vi "Schedule Geode Robot.vi"(6 "max geodes in":u8=24, 7 "max time in":u8=24, 8 "costs in":T1, 9 "data value reference":refnum<data-value>, 10 "stack in":refnum<queue>, 11 "mine in":refnum<class "Mine.lvclass">) -> (0 "costs out":T1, 1 "data value reference":refnum<data-value>, 2 "stack out":refnum<queue>, 3 "mine out":refnum<class "Mine.lvclass">, 4 "max geodes out":u8, 5 "max time out":u8)   [LabVIEW 2023, in "d19.lvlib" / "Mine.lvclass"]
uses:
  Mine.lvclass
  Mine.lvclass/Mine.ctl
  <vilib>/Utility/miscctls.llb/LVMapReplaceAction.ctl
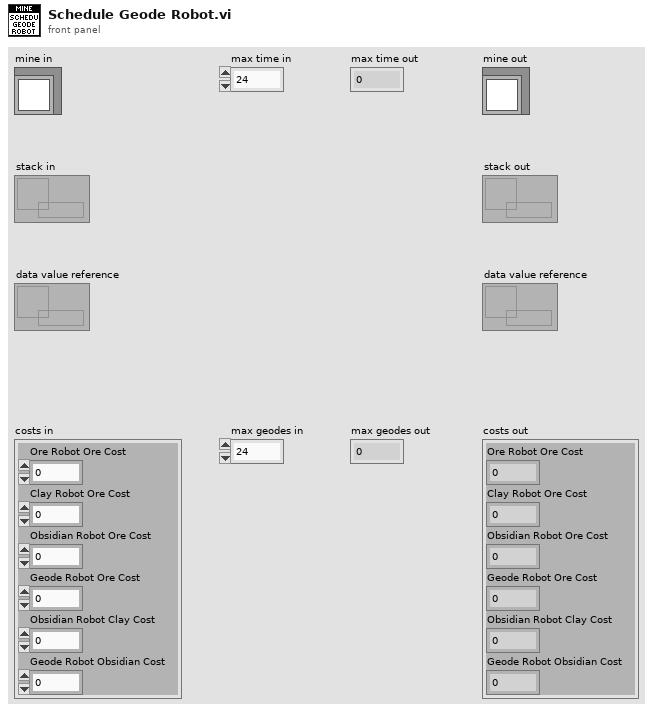
[diagram p1: front panel]
types:
  T1 = cluster{"Ore Robot Ore Cost":u8, "Clay Robot Ore Cost":u8, "Obsidian Robot Ore Cost":u8, "Geode Robot Ore Cost":u8, "Obsidian Robot Clay Cost":u8, "Geode Robot Obsidian Cost":u8}
  T2 = typedef "LVMapReplaceAction.ctl" = enum32{"Modify Entry only if found", "Add or Modify Entry", "Delete Entry"}
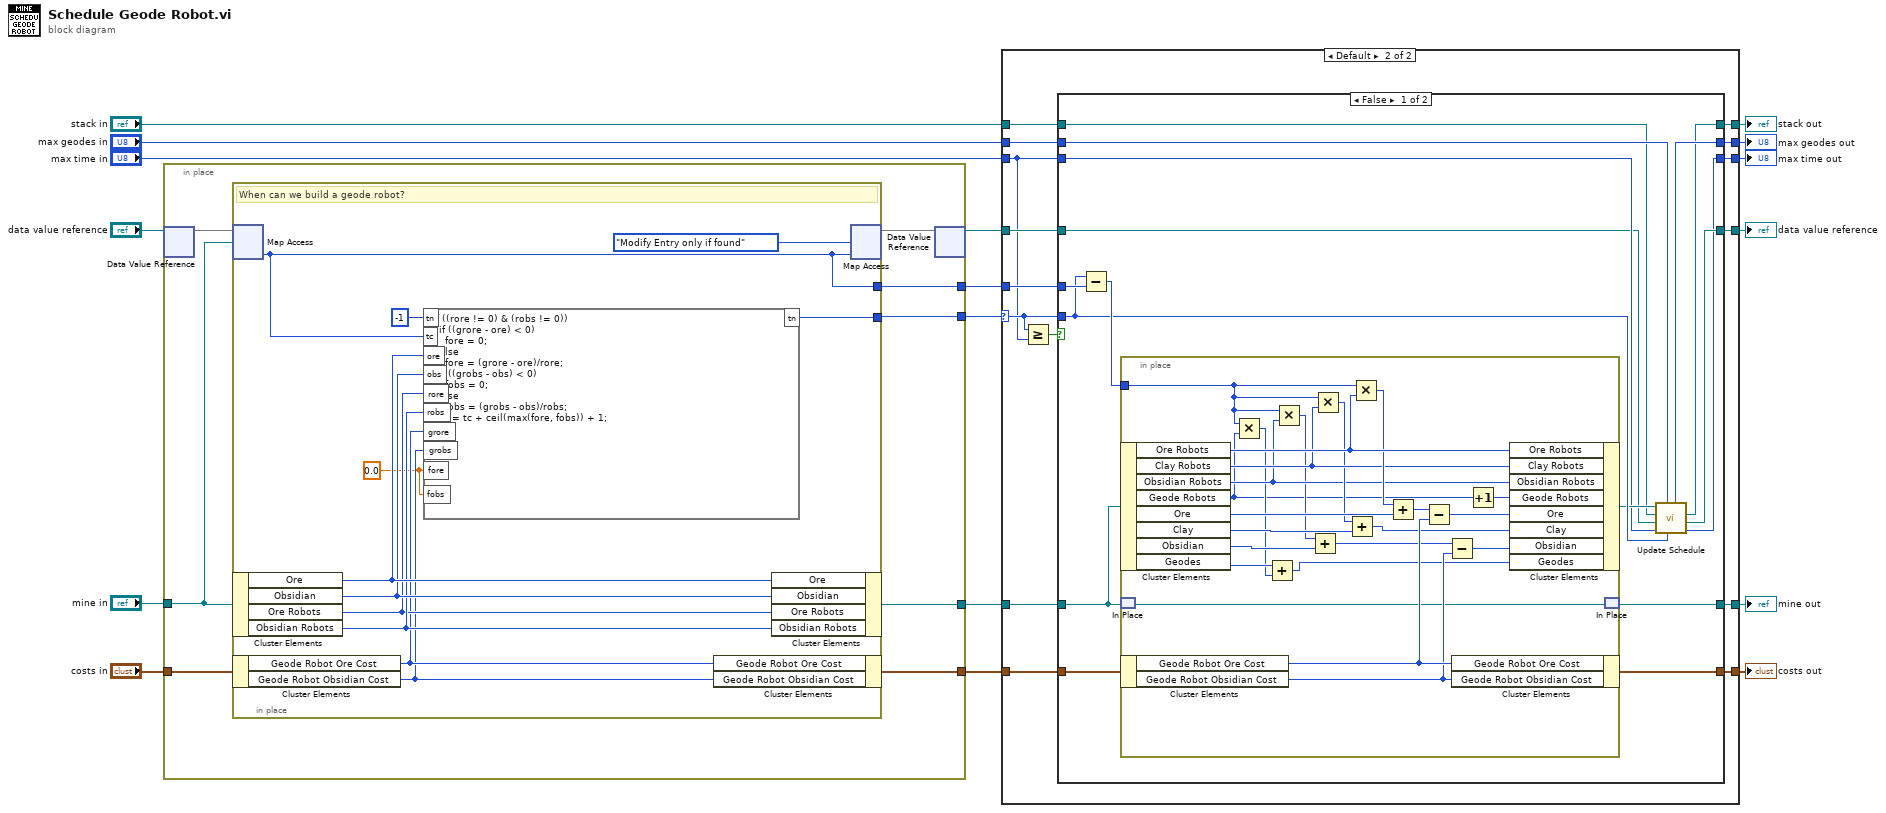
[diagram p0: block diagram]
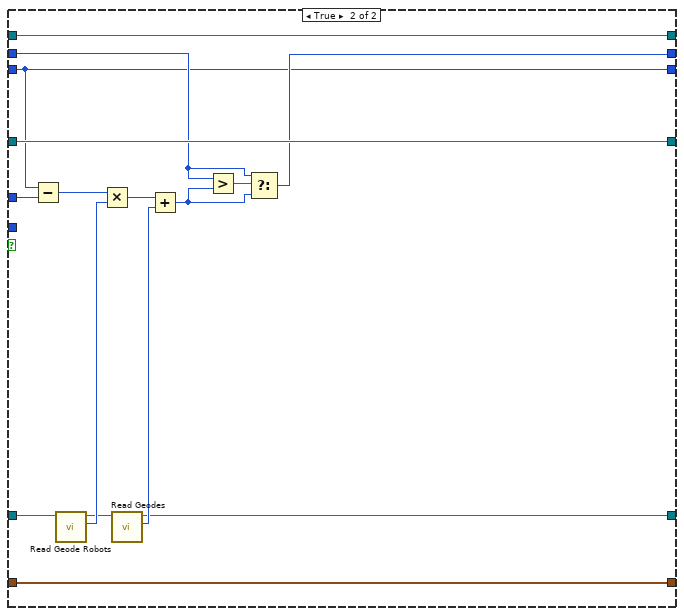
[diagram p3: hidden frame]
diagram:
  n1 = in-place {
    in-place-border: "costs in" -> [w25]
    in-place-border: "mine in" -> [w24]
    in-place-border: [w23] -> w15
    in-place-border: [w22] -> w11
    in-place-border: [w21] -> w10
    in-place-border: [w20] -> w6
    n2 = in-place-dvr #1("data value reference") -> (w19:map{refnum<class "Mine.lvclass">, u8})  [unwired: 1 out]
    n3 = in-place {
      in-place-border: [w28] -> w23
      in-place-border: [w26] -> w20
      w27 = 0.0 ("input variable")
      # "When can we build a geode robot?"
      n4 = in-place-map #2(w19, w24) -> (w26:u8)  [unwired: 1 in, 1 out]
      n5 = in-place-cluster #3(w24) -> ("Ore"=w35:u8, "Obsidian"=w34:u8, "Ore Robots"=w32:u8, "Obsidian Robots"=w33:u8)
      n6 = in-place-cluster #4(w25) -> ("Geode Robot Ore Cost"=w31:u8, "Geode Robot Obsidian Cost"=w30:u8)
      n7 = formula code="if ((rore != 0) & (robs != 0))\n  if ((grore - ore) < 0)\n    fore = 0;\n  else\n    fore = (grore - ore)/rore;\n  if ((grobs - obs) < 0)\n    fobs = 0;\n  else\n    fobs = (grobs - obs)/robs;\n  tn = tc + ceil(max(fore, fobs)) + 1;"("tc"=w26, "grore"=w31, "grobs"=w30, "ore"=w35, "obs"=w34, "rore"=w32, "robs"=w33, "tn"=i8 -1, "fore"=w27, "fobs"=w27) -> ("tn"=w28:i8)
      n8 = in-place-cluster #4("Geode Robot Ore Cost"=w31, "Geode Robot Obsidian Cost"=w30) -> (w22:T1)
      n9 = in-place-cluster #3("Ore"=w35, "Obsidian"=w34, "Ore Robots"=w32, "Obsidian Robots"=w33) -> (w21:refnum<class "Mine.lvclass">)
      n10 = in-place-map #2(w26, LVMapReplaceAction."Modify Entry only if found" ("action")) -> (w18:map{refnum<class "Mine.lvclass">, u8})  [unwired: 2 out]
    }
    n11 = in-place-dvr #1(w18) -> (w1:refnum<data-value>)  [unwired: 1 out]
  }
  n12 = case shown="Default" w15 {
    selector: w15 -> [_ w45]
    tunnel: "stack in" -> [w42 w57]
    tunnel: [w42 w56] -> w13
    tunnel: [w39 w55] -> w12
    tunnel: w11 -> [w37 w54]
    tunnel: w10 -> [w38 w53]
    tunnel: [w37 w52] -> w9
    tunnel: [w38 w51] -> w8
    tunnel: "max time in" -> [w40 w44]
    tunnel: w6 -> [_ w50]
    tunnel: "max geodes in" -> [w41 w49]
    tunnel: [w41 w48] -> w4
    tunnel: [w40 w47] -> w3
    tunnel: w1 -> [w39 w46]
    frame -1 {
    }
    frame Default {
      n13 = Greater Or Equal?(x=w45, y=w44) -> (x >= y?=w43:bool)
      n14 = case shown="False" w43 {
        tunnel: w46 -> [w62 w112]
        tunnel: [w60 w112] -> w55
        tunnel: w57 -> [w61 w111]
        tunnel: [w59 w111] -> w56
        tunnel: w54 -> [w73 w110]
        tunnel: w53 -> [w69 w99]
        tunnel: [w72 w110] -> w52
        tunnel: [w68 w97] -> w51
        tunnel: w44 -> [w63 w106]
        tunnel: w50 -> [w71 w105]
        tunnel: w49 -> [w67 w107]
        tunnel: [w66 w108] -> w48
        tunnel: [w58 w106] -> w47
        tunnel: w45 -> [w65 _]
        frame False {
          n15 = Subtract(x=w65, y=w71) -> (x-y=w70:u8)
          n16 = in-place {
            in-place-border: w70 -> [w78]
            n17 = in-place-cluster #5(w69) -> ("Ore Robots"=w88:u8, "Clay Robots"=w84:u8, "Obsidian Robots"=w82:u8, "Geode Robots"=w76:u8, "Ore"=w96:u8, "Clay"=w91:u8, "Obsidian"=w81:u8, "Geodes"=w90:u8)
            n18 = in-place-match #6(w69) -> (w89:refnum<class "Mine.lvclass">)
            n19 = in-place-cluster #7(w73) -> ("Geode Robot Ore Cost"=w95:u8, "Geode Robot Obsidian Cost"=w94:u8)
            n20 = Multiply(x=w78, y=w76) -> (x*y=w77:u8)
            n21 = Add(x=w90, y=w77) -> (x+y=w75:u8)
            n22 = Multiply(x=w78, y=w82) -> (x*y=w79:u8)
            n23 = Add(x=w79, y=w81) -> (x+y=w80:u8)
            n24 = Multiply(x=w78, y=w84) -> (x*y=w83:u8)
            n25 = Add(x=w83, y=w91) -> (x+y=w86:u8)
            n26 = Multiply(x=w78, y=w88) -> (x*y=w85:u8)
            n27 = Add(x=w85, y=w96) -> (x+y=w87:u8)
            n28 = Subtract(x=w87, y=w95) -> (x-y=w92:u8)
            n29 = Subtract(x=w80, y=w94) -> (x-y=w93:u8)
            n30 = in-place-cluster #7("Geode Robot Ore Cost"=w95, "Geode Robot Obsidian Cost"=w94) -> (w72:T1)
            n31 = Increment(x=w76) -> (x+1=w74:u8)
            n32 = in-place-cluster #5("Ore Robots"=w88, "Clay Robots"=w84, "Obsidian Robots"=w82, "Geode Robots"=w74, "Ore"=w92, "Clay"=w86, "Obsidian"=w93, "Geodes"=w75) -> (w64:refnum<class "Mine.lvclass">)
            n33 = in-place-match #6(w89) -> (w68:refnum<class "Mine.lvclass">)
          }
          n34 = call "Update Schedule.vi"("new time"=w65, "max geodes in"=w67, "max time in"=w63, "map in"=w62, "stack in"=w61, "Mine in"=w64) -> ("max time out"=w58:u8, "map out"=w60:refnum<data-value>, "stack out"=w59:refnum<queue>, "max geodes out"=w66:u8)  [unwired: 1 in, 1 out]
        }
        frame True {
          n35 = Subtract(x=w106, y=w105) -> (x-y=w104:u8)
          n36 = call "Read Geode Robots.vi"("Mine in"=w99) -> ("Geode Robots"=w103:u8, "Mine out"=w98:refnum<class "Mine.lvclass">)  [unwired: 9 in]
          n37 = Multiply(x=w104, y=w103) -> (x*y=w100:u8)
          n38 = call "Read Geodes.vi"("Mine in"=w98) -> ("Geodes"=w102:u8, "Mine out"=w97:refnum<class "Mine.lvclass">)  [unwired: 9 in]
          n39 = Add(x=w100, y=w102) -> (x+y=w101:u8)
          n40 = Greater?(x=w107, y=w101) -> (0:w109:bool)
          n41 = Select(t=w107, s=w109, f=w101) -> (s? t:f=w108:u8)
        }
      }
    }
  }
  "stack out" <- w13
  "data value reference" <- w12
  "costs out" <- w9
  "mine out" <- w8
  "max geodes out" <- w4
  "max time out" <- w3
